vi "Agilent 681x Acquire Current Measurement.vi"() -> ()   [LabVIEW 2019]
doc: "Shows how to acquire a current measurement."
uses:
  <instrlib>/Agilent 681x Series/Public/Data/Read Single Measurement (Current).vi
  <instrlib>/Agilent 681x Series/Agilent 681x Series.lvlib
panel:
  in  "Sample Spacing (25 us)":dbl=2.5e-05 format="%^.2g"
  in  "Sense Source (0: Internal)":u16(ring) items=["Internal", "External"]
  in  "Output Frequency (60 Hz)":dbl=60.0 format="%#.4g"
  in  "Voltage Amplitude (1.0 V)":dbl=1.0 format="%#.4g"
  in  "Relative Trigger Samples (0)":i32
  in  "Output Waveform Type (0: Sinusoid)":u16(ring) items=["Sinusoid", "Square", "Clipped Sinusoid", "User Specified"]
  out "Peak Current":dbl
  out "AC + DC RMS Current":dbl
  out "AC RMS Current":dbl
  out "DC Current":dbl
  in  "Maximum Time (10000 ms)":i32=10000
  in  "User-Specified Output Waveform Name":string
  in  "Serial Configuration":T1={"Baud Rate"=9600, "Parity"=0, "Data Bits"=8} {"Data Bits" items=["7"=7, "8"=8]; "Parity" items=["None", "Odd", "Even", "Mark", "Space"]; "Baud Rate" items=["300"=300, "600"=600, "1200"=1200, "2400"=2400, "4800"=4800, "9600"=9600]}
  in  "VISA resource name":refnum<visa-resource-name>
  # "VI para definir:\n    1) tensão de saída da fonte \n    2) forma de onda,\n    3) frequência da onda. \n    4) medir valores de corrente elétrica aplicados pela fonte."
  # "(c) 2008-2021 National Instruments Corp.  ALL RIGHTS RESERVED."
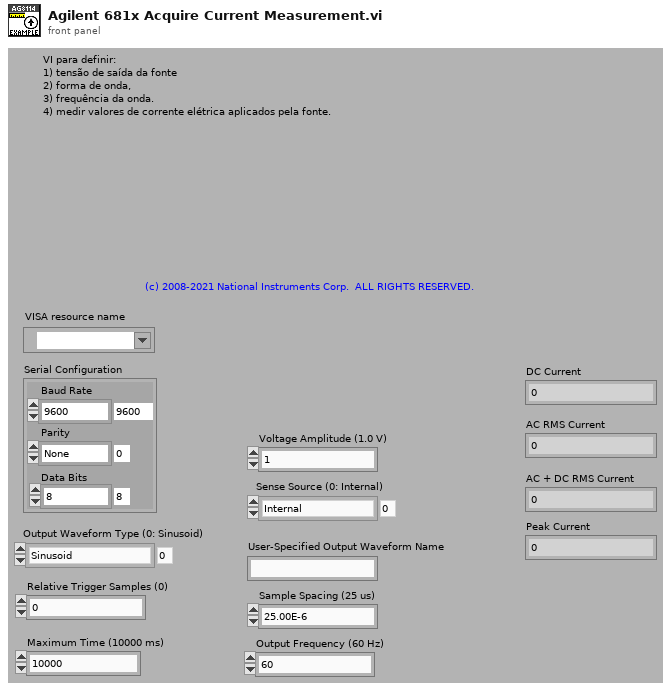
[diagram p1: front panel]
types:
  T1 = cluster{"Baud Rate":u32, "Parity":u16, "Data Bits":u16}
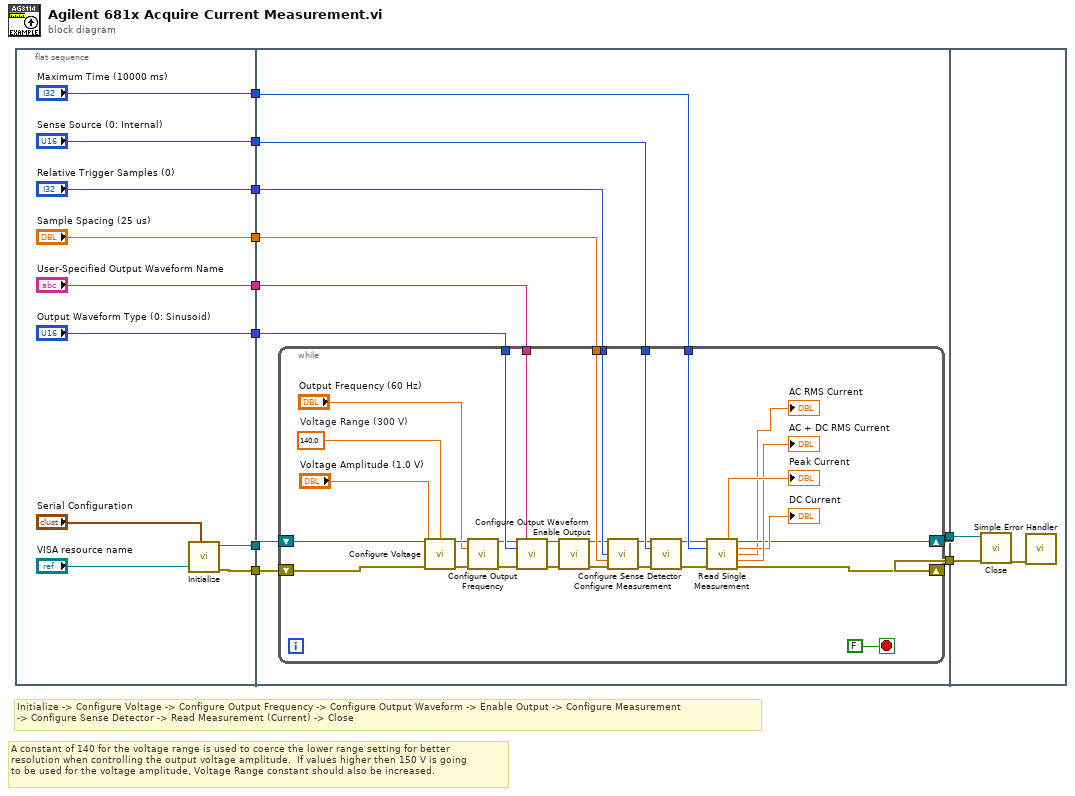
[diagram p0: block diagram]
diagram:
  # "Initialize -> Configure Voltage -> Configure Output Frequency -> Configure Output Waveform -> Enable Output -> Configure Measurement\n-> Configure Sense Detector -> Read Measurement (Current) -> Close"
  # "A constant of 140 for the voltage range is used to coerce the lower range setting for better\nresolution when controlling the output voltage amplitude.  If values higher then 150 V is going\nto be used for the voltage amplitude, Voltage Range constant should also be increased."
  n1 = flat-sequence {
    tunnel: ["Maximum Time (10000 ms)"] -> w10
    tunnel: ["Sense Source (0: Internal)"] -> w9
    tunnel: ["Relative Trigger Samples (0)"] -> w8
    tunnel: ["Sample Spacing (25 us)"] -> w7
    tunnel: ["User-Specified Output Waveform Name"] -> w6
    tunnel: ["Output Waveform Type (0: Sinusoid)"] -> w5
    tunnel: [w14] -> w4
    tunnel: [w13] -> w3
    tunnel: w10 -> [w30]
    tunnel: w9 -> [w29]
    tunnel: w8 -> [w28]
    tunnel: w7 -> [w27]
    tunnel: w6 -> [w26]
    tunnel: w5 -> [w25]
    tunnel: w4 -> [w24]
    tunnel: w3 -> [w23]
    tunnel: [w22] -> w2
    tunnel: [w21] -> w1
    tunnel: w2 -> [w63]
    tunnel: w1 -> [w62]
    frame #0 {
      n2 = call <instrlib>:"Initialize.vi"("Serial Configuration"="Serial Configuration", "VISA resource name"="VISA resource name") -> ("error out"=w14:errorcluster, "VISA resource name out"=w13:refnum<visa-resource-name>)  [unwired: 8 in]
    }
    frame #1 {
      n3 = while {
        tunnel: w30 -> [w60]
        tunnel: w29 -> [w59]
        tunnel: w28 -> [w58]
        tunnel: w27 -> [w57]
        tunnel: w26 -> [w56]
        tunnel: w25 -> [w55]
        shift-right: [w37] -> w22
        shift-left: w24 -> [w54]
        shift-right: [w36] -> w21
        shift-left: w23 -> [w53]
        stop <- FALSE stop-if-true
        w33 = 140.0  # Voltage Range (300 V)
        n4 = call <instrlib>:"Configure Voltage.vi"("VISA resource name"=w53, "Voltage Range (300 V)"=w33, "Voltage Amplitude (1.0 V)"="Voltage Amplitude (1.0 V)", "error in (no error)"=w54) -> ("VISA resource name out"=w49:refnum<visa-resource-name>, "error out"=w48:errorcluster)  [unwired: 10 in]
        n5 = call <instrlib>:"Configure Output Frequency.vi"("VISA resource name"=w49, "Output Frequency (60 Hz)"="Output Frequency (60 Hz)", "error in (no error)"=w48) -> ("VISA resource name out"=w41:refnum<visa-resource-name>, "error out"=w40:errorcluster)  [unwired: 11 in]
        n6 = call <instrlib>:"Configure Output Waveform.vi"("VISA resource name"=w41, "User-Specified Output Waveform Name"=w56, "Output Waveform Type (0: Sinusoid)"=w55, "error in (no error)"=w40) -> ("VISA resource name out"=w39:refnum<visa-resource-name>, "error out"=w38:errorcluster)  [unwired: 10 in]
        n7 = call <instrlib>:"Enable Output.vi"("VISA resource name"=w39, "error in (no error)"=w38) -> ("VISA resource name out"=w42:refnum<visa-resource-name>, "error out"=w43:errorcluster)  [unwired: 12 in]
        n8 = call <instrlib>:"Configure Measurement.vi"("VISA resource name"=w42, "Relative Trigger Samples (0)"=w58, "Sample Spacing (25 us)"=w57, "error in (no error)"=w43) -> ("VISA resource name out"=w44:refnum<visa-resource-name>, "error out"=w45:errorcluster)  [unwired: 10 in]
        n9 = call <instrlib>:"Configure Sense Detector.vi"("VISA resource name"=w44, "Sense Source (0: Internal)"=w59, "error in (no error)"=w45) -> ("VISA resource name out"=w47:refnum<visa-resource-name>, "error out"=w46:errorcluster)  [unwired: 11 in]
        n10 = call-poly <instrlib>:"Read Single Measurement.vi"("VISA resource name"=w47, "Maximum Time (10000 ms)"=w60, "error in (no error)"=w46) -> ("Peak Current"=→"Peak Current":dbl, "VISA resource name out"=w36:refnum<visa-resource-name>, "DC Current"=→"DC Current":dbl, "AC RMS Current"=→"AC RMS Current":dbl, "AC + DC RMS Current"=→"AC + DC RMS Current":dbl, "error out"=w37:errorcluster)  [unwired: 7 in]
      }
    }
    frame #2 {
      n11 = call <instrlib>:"Close.vi"("error in (no error)"=w63, "VISA resource name"=w62) -> ("error out"=w61:errorcluster)  [unwired: 9 in]
      n12 = call <vilib>:"Simple Error Handler.vi"("error in (no error)"=w61) -> ()  [unwired: 4 in, 5 out]
    }
  }
